vi "update_dichroic_mirror.vi"(4 "error in (no error)":errorcluster, 5 "commit?":bool, 6 "dichroic mirror #":u16, 7 "VISA resource name":refnum<visa-resource-name>) -> (0 "error out":errorcluster, 1 "update COM error status":bool, 2 "cmd string":string, 3 "VISA resource name out":refnum<visa-resource-name>)   [LabVIEW 2016]
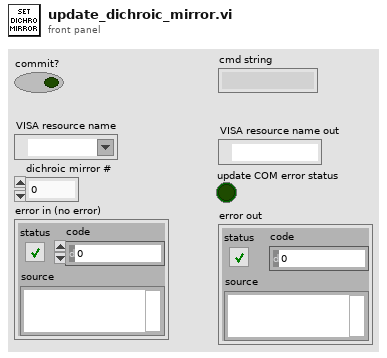
[diagram p1: front panel]
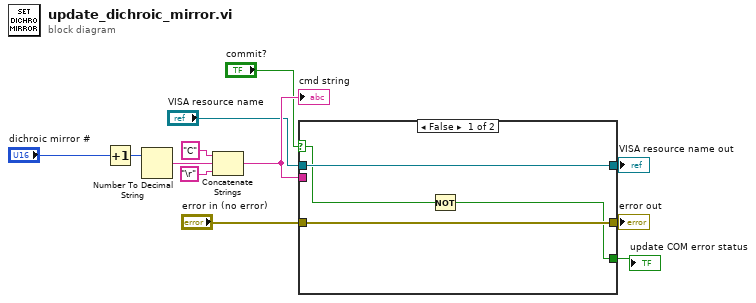
[diagram p0: block diagram]
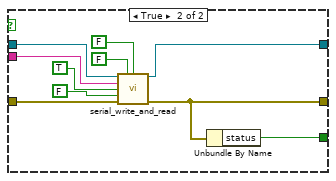
[diagram p2: hidden frame]
diagram:
  n1 = Increment(x="dichroic mirror #") -> (x+1=w7:u16)
  n2 = Number To Decimal String(number=w7) -> (decimal integer string=w12:string)  [unwired: 1 in]
  n3 = Concatenate Strings("C" ("string"), w12, "\r") -> (w9:string)
  "cmd string" <- w9
  n4 = case shown="False" "commit?" {
    selector: "commit?" -> [w14 _]
    tunnel: w9 -> [_ w24]
    tunnel: [w15 w18] -> w8
    tunnel: "VISA resource name" -> [w16 w26]
    tunnel: [w16 w19] -> w4
    tunnel: "error in (no error)" -> [w15 w25]
    tunnel: [w13 w17] -> w1
    frame False {
      n5 = Not(x=w14) -> (.not. x?=w13:bool)
    }
    frame True {
      n6 = call "serial_write_and_read.vi"("port name in"=w26, "reconnect?"=FALSE, "disconnect?"=FALSE, "write buffer"=w24, "do writing?"=TRUE, "expecting response?"=FALSE, "error in"=w25) -> ("port name out"=w19:refnum<visa-resource-name>, "error out"=w18:errorcluster)  [unwired: 6 in, 1 out]
      n7 = Unbundle By Name(w18) -> ("status"=w17:bool)
    }
  }
  "error out" <- w8
  "VISA resource name out" <- w4
  "update COM error status" <- w1
